vi "AI Test.vi"() -> ()   [LabVIEW 2021]
uses:
  <vilib>/DAQmx/read.llb/DAQmx Read (Analog 1D Wfm NChan NSamp).vi
  <vilib>/DAQmx/create/channels.llb/DAQmx Create Channel (AI-Voltage-Basic).vi
  <vilib>/DAQmx/configure/timing.llb/DAQmx Timing (Sample Clock).vi
  <vilib>/DAQmx/miscellaneous.llb/DAQmx Fill In Error Info.vi
  <resource>/objmgr/daqmx.rc
panel:
  out "data string":string
  out "Waveform Graph":waveform(dbl)[](graph)
  out "Waveform Chart":waveform(dbl)[](graph)
  in  "active edge":i32(ring)=10280 items=["Rising"=10280, "Falling"=10171]
  in  "source":tag
  in  "rate":dbl=1000.0 format="%0.2f"
  in  "samples per channel":i32=1000
  in  "sample mode":i32(ring)=10178 items=["Finite Samples"=10178, "Continuous Samples"=10123, "Hardware Timed Single Point"=12522]
  in  "minimum value":dbl=-5.0 format="%#_13g"
  in  "maximum value":dbl=5.0 format="%#_13g"
  in  "units":i32(ring)=10348 items=["Volts"=10348, "From Custom Scale"=10065]
  in  "physical channels":tag
  out "data":waveform(dbl)[](array[waveform])
  out "AI.PhysicalChans":tag[](array[tag])
  in  "Stop":bool
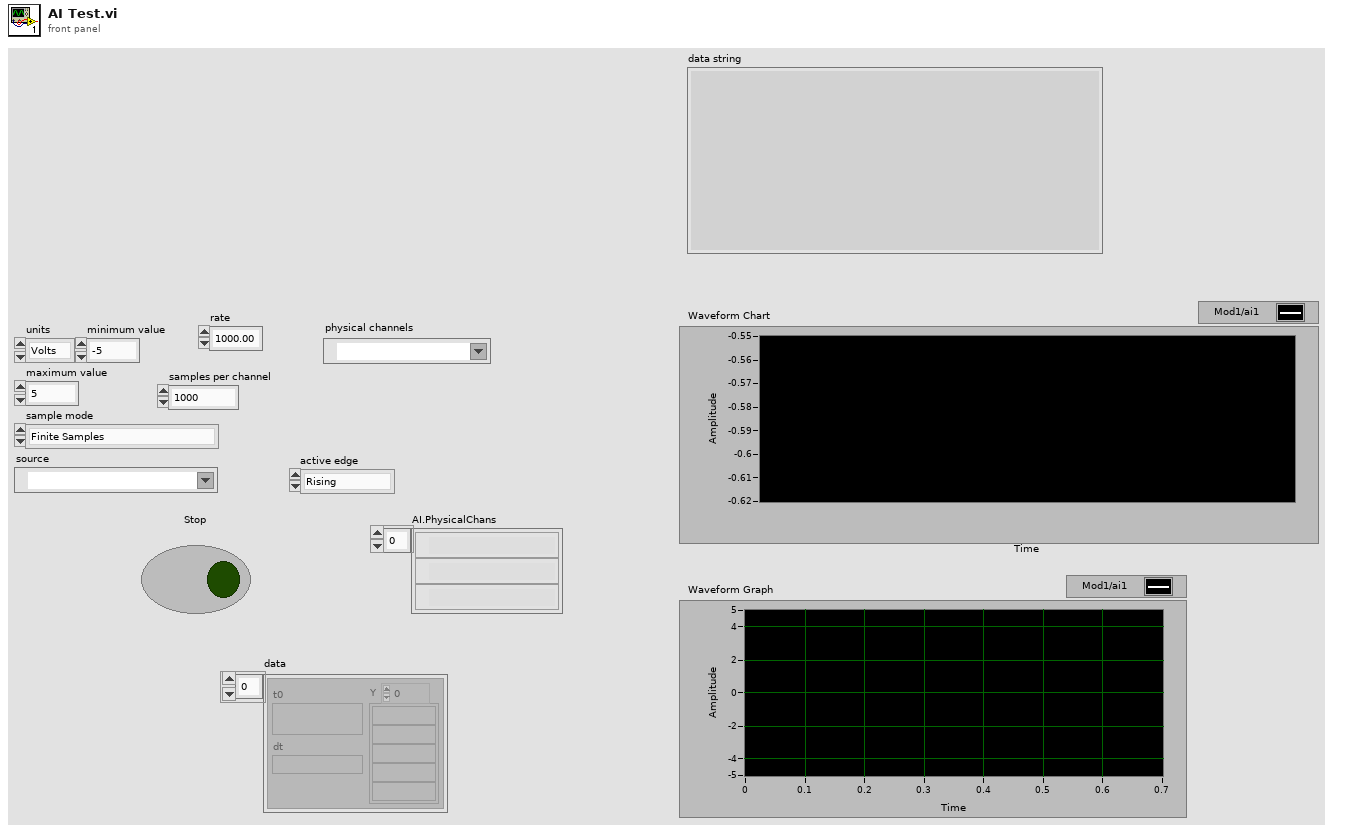
[diagram p1: front panel]
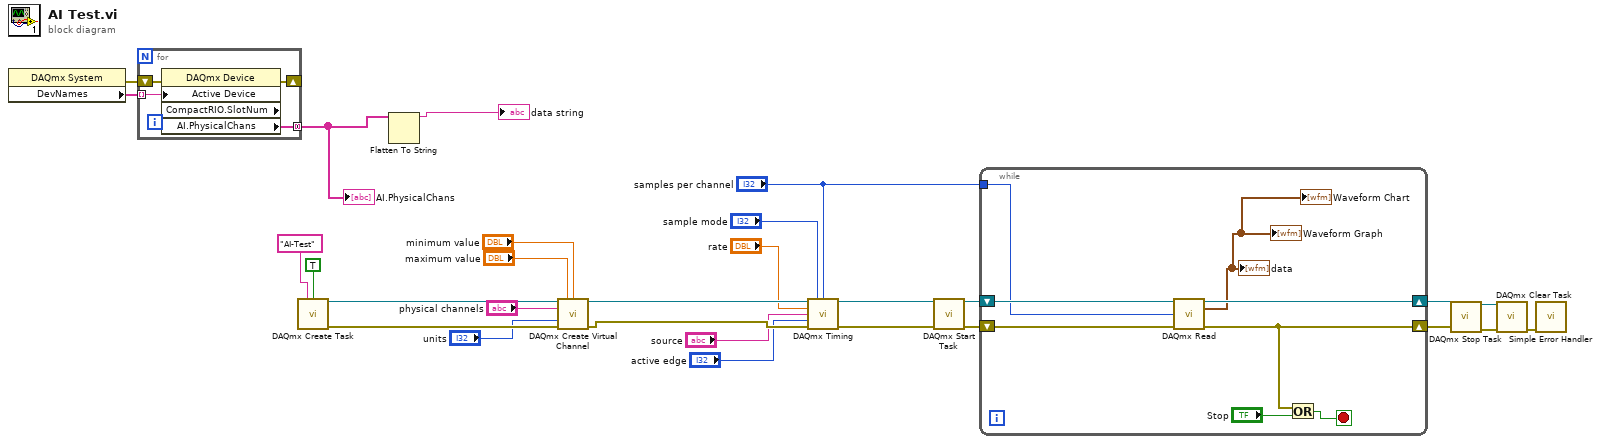
[diagram p0: block diagram]
diagram:
  n1 = property class="DAQmx System"() -> (error out=w23:errorcluster, "DevNames"=w28:tag[])  [unwired: 2 in, 1 out]
  n2 = for {
    tunnel: w28 -> [w32] mode=indexing
    shift-right: [w31] -> _
    shift-left: w23 -> [w30]
    tunnel: [w29] -> w2 mode=concatenating
    n3 = property class="DAQmx Device" props=["Active Device", "CompactRIO.SlotNum", "AI.PhysicalChans"](error in=w30, "Active Device"=w32) -> (error out=w31:errorcluster, "AI.PhysicalChans"=w29:tag[])  [unwired: 1 in, 2 out]
  }
  "AI.PhysicalChans" <- w2
  n4 = call <vilib>:"DAQmx Create Task.vi"("new task name"="AI-Test", "auto cleanup"=TRUE) -> ("task out"=w24:refnum<k21>, "error out"=w25:errorcluster)  [unwired: 12 in]
  n5 = Flatten To String(anything=w2) -> (data string=→"data string":string)  [unwired: 3 in, 2 out]
  n6 = call-poly <vilib>:"DAQmx Create Virtual Channel.vi"("task in"=w24, "maximum value"="maximum value", "minimum value"="minimum value", "physical channels"="physical channels", "units"="units", "error in"=w25) -> ("task out"=w9:refnum<k21>, "error out"=w11:errorcluster)  [unwired: 8 in]
  n7 = call-poly <vilib>:"DAQmx Timing.vi"("task/channels in"=w9, "sample mode"="sample mode", "samples per channel"="samples per channel", "rate"="rate", "source"="source", "active edge"="active edge", "error in"=w11) -> ("task out"=w8:refnum<k21>, "error out"=w10:errorcluster)  [unwired: 7 in]
  n8 = call <vilib>:"DAQmx Start Task.vi"("task/channels in"=w8, "error in"=w10) -> ("task out"=w22:refnum<k21>, "error out"=w21:errorcluster)  [unwired: 12 in]
  n9 = while {
    shift-right: [w35] -> w17
    shift-left: w22 -> [w38]
    shift-right: [w36] -> w20
    shift-left: w21 -> [w37]
    tunnel: "samples per channel" -> [w34]
    stop <- w39 stop-if-true
    n10 = call-poly <vilib>:"DAQmx Read.vi"("task/channels in"=w38, "number of samples per channel"=w34, "error in"=w37) -> ("task out"=w35:refnum<k21>, "data"=→"data" →"Waveform Chart" →"Waveform Graph":waveform(dbl)[], "error out"=w36:errorcluster)  [unwired: 10 in]
    n11 = Or(x=w36, y="Stop") -> (x .or. y?=w39:bool)
  }
  n12 = call <vilib>:"DAQmx Stop Task.vi"("task/channels in"=w17, "error in"=w20) -> ("task out"=w16:refnum<k21>, "error out"=w19:errorcluster)  [unwired: 12 in]
  n13 = call <vilib>:"DAQmx Clear Task.vi"("task in"=w16, "error in"=w19) -> ("error out"=w18:errorcluster)  [unwired: 13 in]
  n14 = call <vilib>:"Simple Error Handler.vi"("error in (no error)"=w18) -> ()  [unwired: 4 in, 5 out]
